vi "Show Hide (Label).vi"(5 "Invert? [F]":bool, 7 "Regex? [F]":bool, 8 "error in (no error)":errorcluster, 9 "Show? [T]":bool=TRUE, 10 "Label":string, 11 "MMI Scaling in":refnum<class "Interaction By Refererence.lvclass">) -> (0 "error out":errorcluster, 2 "Match?":bool, 3 "MMI Scaling out":refnum<class "Interaction By Refererence.lvclass">)   [LabVIEW 2021, in "Interaction By Refererence.lvclass"]
uses:
  Interaction By Refererence.lvclass
  Interaction By Refererence.lvclass/Interaction By Refererence.ctl
  IContainer/Interaction/Interaction.lvclass
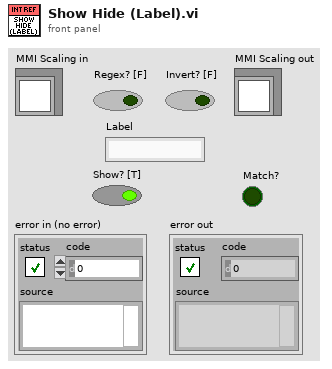
[diagram p1: front panel]
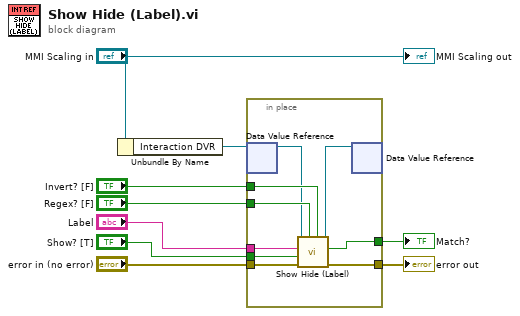
[diagram p0: block diagram]
diagram:
  n1 = Unbundle By Name("MMI Scaling in") -> ("Interaction DVR"=w2:refnum<data-value>)
  n2 = in-place {
    in-place-border: [w18] -> w9
    in-place-border: "Invert? [F]" -> [w17]
    in-place-border: "Regex? [F]" -> [w16]
    in-place-border: "error in (no error)" -> [w15]
    in-place-border: "Show? [T]" -> [w14]
    in-place-border: "Label" -> [w13]
    in-place-border: [w10] -> w1
    n3 = in-place-dvr #1(w2) -> (w12:refnum<class "Interaction.lvclass">)  [unwired: 1 out]
    n4 = call-dynamic "Show Hide (Label).vi"("Invert? [F]"=w17, "Regex? [F]"=w16, "error in (no error)"=w15, "Show? [T]"=w14, "Label"=w13, "MMI Scaling in"=w12) -> ("error out"=w18:errorcluster, "Match?"=w10:bool, "MMI Scaling out"=w11:refnum<class "Interaction.lvclass">)  [unwired: 3 in]
    n5 = in-place-dvr #1(w11) -> ()  [unwired: 2 out]
  }
  "error out" <- w9
  "Match?" <- w1
  "MMI Scaling out" <- "MMI Scaling in"
